vi "Set Conn Pane Recommended to Required.vi"(8 "error in (no error)":errorcluster, 11 "VI Ref":refnum<vi>) -> (0 "error out":errorcluster, 2 "Save?":bool, 3 "VI Ref out":refnum<vi>)   [LabVIEW 2020, in "Code Cleanup.lvlib"]
uses:
  Code Cleanup.lvlib
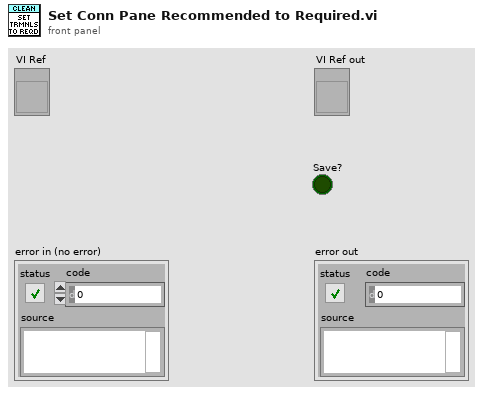
[diagram p1: front panel]
types:
  T1 = enum16{"Invalid Wire Rule", "Required", "Recommended", "Optional", "Dynamic Dispatch"}[]
  T2 = enum16{"Invalid Wire Rule", "Required", "Recommended", "Optional", "Dynamic Dispatch"}
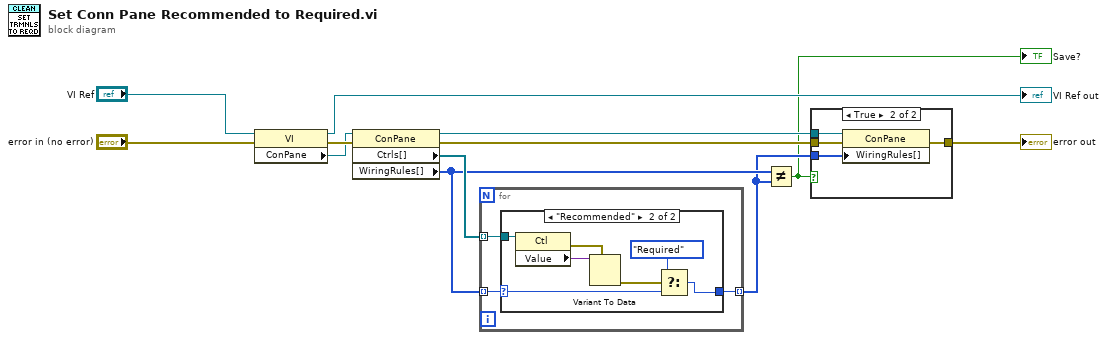
[diagram p0: block diagram]
diagram:
  n1 = property class="VI"(reference="VI Ref", error in="error in (no error)") -> (reference out=→"VI Ref out":refnum<vi>, error out=w11:errorcluster, "ConPane"=w6:refnum<vi>)
  n2 = property class="ConPane"(reference=w6, error in=w11) -> (reference out=w9:refnum<vi>, error out=w10:errorcluster, "Ctrls[]"=w7:refnum<vi>[], "WiringRules[]"=w3:T1)
  n3 = for {
    tunnel: w3 -> [w15] mode=indexing
    tunnel: [w14] -> w2 mode=indexing
    tunnel: w7 -> [w13] mode=indexing
    n4 = case shown="\"Recommended\"" w15 {
      selector: w15 -> [w16 w19]
      tunnel: [w16 w18] -> w14
      tunnel: w13 -> [_ w17]
      frame Default {
      }
      frame "Recommended" {
        n5 = property class="Ctl"(reference=w17) -> (error out=w22:errorcluster, "Value"=w23:variant)  [unwired: 1 in, 1 out]
        n6 = Variant To Data(type=w22, Variant=w23) -> (error out=w21:errorcluster)  [unwired: 1 in, 1 out]
        n7 = Select(t=T2."Required" ("Wire Rule"), s=w21, f=w19) -> (s? t:f=w18:T2)
      }
    }
  }
  n8 = Not Equal?(x=w3, y=w2) -> (x != y?=w1:bool)
  "Save?" <- w1
  n9 = case shown="True" w1 {
    tunnel: w10 -> [w24 w28]
    tunnel: w9 -> [_ w27]
    tunnel: w2 -> [_ w26]
    tunnel: [w24 w25] -> w8
    frame False {
    }
    frame True {
      n10 = property class="ConPane"(reference=w27, error in=w28, "WiringRules[]"=w26) -> (error out=w25:errorcluster)  [unwired: 1 out]
    }
  }
  "error out" <- w8
